vi "RSZVB Get IMOD Tone Distance.vi"(8 "error in (no error)":errorcluster {"code" format="%.0x"}, 10 "Channel (1)":i32=1, 11 "VISA session":refnum<visa-resource-name>) -> (0 "error out":errorcluster {"code" format="%.0x"}, 1 "Tone Distance":dbl format="%^.3e", 3 "dup VISA session":refnum<visa-resource-name>)   [LabVIEW 2011]
doc: "This VI returns the tone distance (frequency offset) between the upper and the lower tone.\n\nNote(s):\n\n(1) This VI is not available for R&S ZVB instrument.\n\nRemote-control command(s):\n[SENSe<Ch>:]FREQuency:IMODulation:TDIStance?"
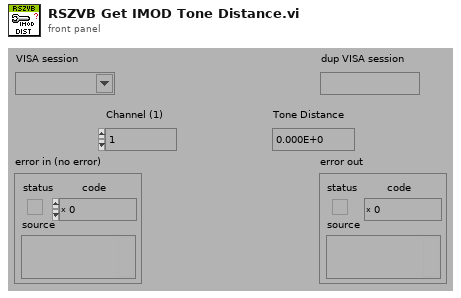
[diagram p1: front panel]
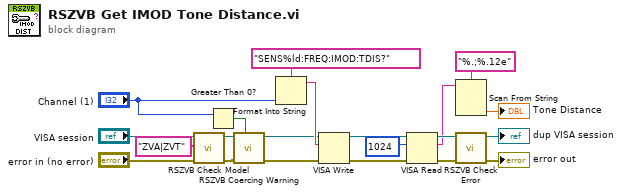
[diagram p0: block diagram]
diagram:
  n1 = call "RSZVB Check Model.vi"("error in (no error)"="error in (no error)", "Model"="ZVA|ZVT", "VISA session"="VISA session") -> ("error out"=w3:errorcluster, "dup VISA session"=w2:refnum<visa-resource-name>)  [unwired: 7 in]
  n2 = Greater Than 0?(x="Channel (1)") -> (x > 0?=w18:bool)
  n3 = call "RSZVB Coercing Warning.vi"("In Range?"=w18, "error in (no error)"=w3, "VISA session"=w2) -> ("error out"=w20:errorcluster, "dup VISA session"=w19:refnum<visa-resource-name>)  [unwired: 7 in]
  n4 = Format Into String(format string="SENS%ld:FREQ:IMOD:TDIS?", "Channel (1)") -> (resulting string=w21:string)  [unwired: 2 in, 1 out]
  n5 = VISA Write(VISA resource name=w19, write buffer=w21, error in (no error)=w20) -> (VISA resource name out=w15:refnum<visa-resource-name>, error out=w14:errorcluster)  [unwired: 1 out]
  n6 = VISA Read(VISA resource name=w15, byte count=u32 1024 ("byte count (0)"), error in (no error)=w14) -> (VISA resource name out=w12:refnum<visa-resource-name>, read buffer=w6:string, error out=w11:errorcluster)  [unwired: 1 out]
  n7 = Scan From String(format string="%.;%.12e", input string=w6) -> (output 1=→"Tone Distance":dbl)  [unwired: 3 in, 3 out]
  n8 = call "RSZVB Check Error.vi"("error in (no error)"=w11, "VISA session"=w12) -> ("error out"=→"error out":errorcluster, "dup VISA session"=→"dup VISA session":refnum<visa-resource-name>)  [unwired: 8 in]
